vi "Write Single Holding Register1.vi"(7 "Unit_ID":T1={"Protocol ID"=0, "Unit ID"=1}, 8 "error in (no error)":errorcluster, 9 "holding register value":u16, 10 "address":u16, 11 "Modbus master in":refnum<class "TCP.lvclass">) -> (0 "error out":errorcluster, 3 "Modbus master out":refnum<class "TCP.lvclass">)   [LabVIEW 2019, in "NI_modbus_upd.lvlib"]
doc: "Writes a value to a single holding register."
uses:
  NI_modbus_upd.lvlib
  TCP/TCP.lvclass
  Ctl/Unit_ID.ctl
  TCP/TCP.lvclass/TCP.ctl
  Function code mismatch error1.vi
  Error Generator1.vi
  Read ADU Packet Master.vi
  Write ADU Packet Master.vi
  Modbus Data Unit (PDU)/Construct PDU1.vi
  Modbus Data Unit (PDU)/Unflatten to PDU1.vi
  TCP/Protocol Read.vi
  TCP/Protocol Write.vi
  <vilib>/Utility/error.llb/Error Cluster From Error Code.vi
  Modbus Data Unit (PDU)/Deconstruct PDU1.vi
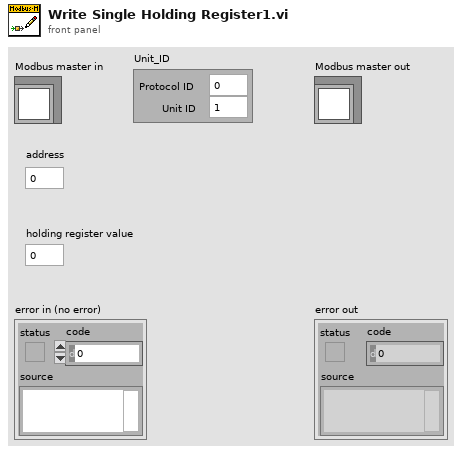
[diagram p1: front panel]
types:
  T1 = typedef "NI_modbus_upd.lvlib/Unit_ID.ctl" = cluster{"Protocol ID":u16, "Unit ID":u8}
  T2 = typedef "NI_modbus_upd.lvlib/MB Modbus Data Unit.ctl" = cluster{"function":T3, "Data":u8[]}
  T3 = typedef "NI_modbus_upd.lvlib/Function.ctl" = u8
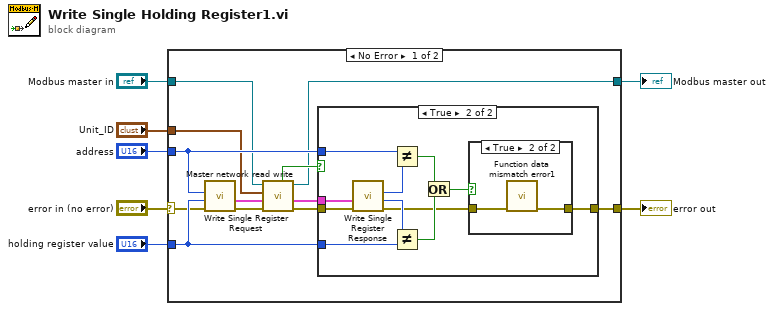
[diagram p0: block diagram]
diagram:
  n1 = case shown="No Error" "error in (no error)" {
    selector: "error in (no error)" -> [w13 w35]
    tunnel: "Modbus master in" -> [w9 w36]
    tunnel: [w10 w36] -> w5
    tunnel: [w18 w35] -> w4
    tunnel: "address" -> [w17 _]
    tunnel: "holding register value" -> [w16 _]
    tunnel: "Unit_ID" -> [w8 _]
    frame No Error {
      n2 = call "Write Single Register Request.vi"("error in (no error)"=w13, "register value"=w16, "starting address"=w17) -> ("error out"=w19:errorcluster, "Modbus Data Unit out"=w12:T2)  [unwired: 7 in]
      n3 = call "Master network read write.vi"("error in (no error)"=w19, "Modbus Data Unit"=w12, "Unit_ID"=w8, "TCP in"=w9) -> ("error out"=w15:errorcluster, "Modbus data unit out"=w11:T2, "TCP out"=w10:refnum<class "TCP.lvclass">, "PDU valid?"=w14:bool)  [unwired: 4 in]
      n4 = case shown="True" w14 {
        tunnel: [w20 w28] -> w18
        tunnel: w17 -> [_ w23]
        tunnel: w16 -> [_ w27]
        tunnel: w15 -> [w20 w25]
        tunnel: w11 -> [_ w21]
        frame False {
        }
        frame True {
          n5 = call "Write Single Register Response.vi"("error in (no error)"=w25, "Modbus Data Unit in"=w21) -> ("error out"=w24:errorcluster, "number of coils"=w26:u16, "address"=w22:u16)  [unwired: 7 in]
          n6 = Not Equal?(x=w23, y=w22) -> (x != y?=w30:bool)
          n7 = Not Equal?(x=w26, y=w27) -> (x != y?=w31:bool)
          n8 = Or(x=w30, y=w31) -> (x .or. y?=w29:bool)
          n9 = case shown="True" w29 {
            tunnel: [w32 w34] -> w28
            tunnel: w24 -> [w32 w33]
            frame False {
            }
            frame True {
              n10 = call "Function data mismatch error1.vi"("error in (no error)"=w33) -> ("error out"=w34:errorcluster)  [unwired: 10 in]
            }
          }
        }
      }
    }
    frame Error {
    }
  }
  "error out" <- w4
  "Modbus master out" <- w5
